vi "IMAQ subtract background.vi"(7 "FakeCamera in":refnum<class "Point Grey Camera.lvclass">, 8 "error in (no error)":errorcluster, 11 "Image in":T1) -> (0 "error out":errorcluster, 1 "Intensity Graph":u16[][](graph), 2 "Line Graph 2":cluster{"x0":sgl, "dx":sgl, "Pixels Line":sgl[]} {"dx" format="%.2f"; "x0" format="%.2f"}, 3 "Refnum out":T1, 4 "Line Graph":cluster{"x0":sgl, "dx":sgl, "Pixels Line":sgl[]} {"dx" format="%.2f"; "x0" format="%.2f"}, 5 "FakeCamera out":refnum<class "Point Grey Camera.lvclass">)   [LabVIEW 2020, in "Point Grey Camera.lvclass"]
uses:
  Point Grey Camera.lvclass
  IMAQ Image.ctl
  Point Grey Camera.lvclass/Point Grey Camera.ctl
  NI_Vision_Development_Module.lvlib
  NI_AALBase.lvlib
panel:
  out "create BG":u32
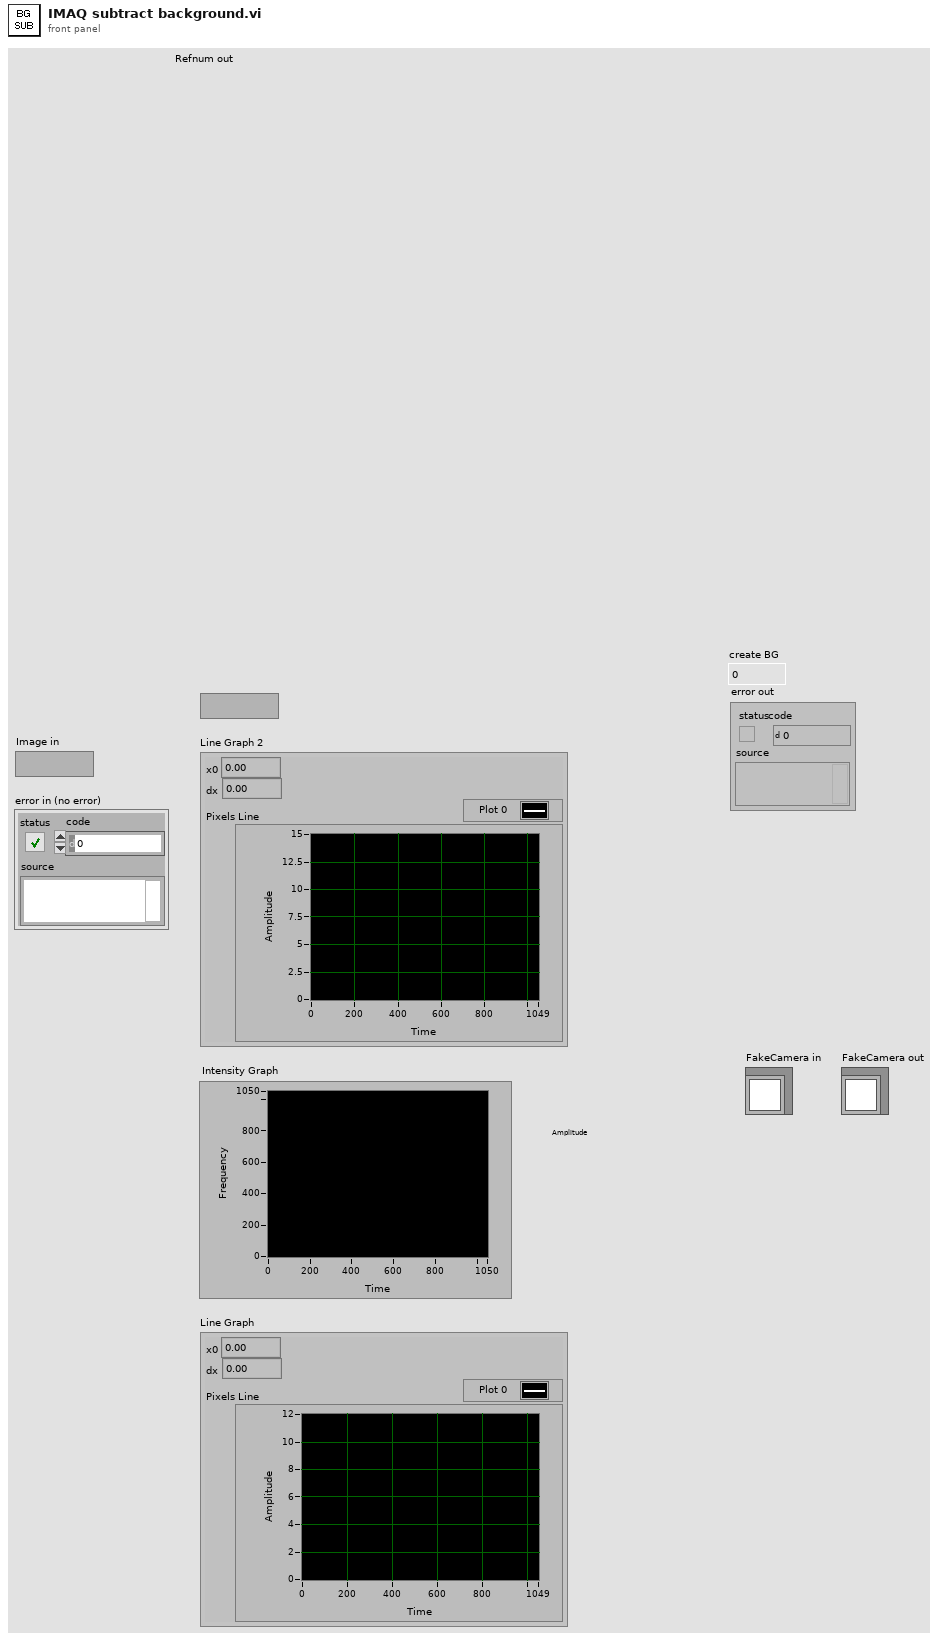
[diagram p1: front panel]
types:
  T1 = typedef "IMAQ Image.ctl" = refnum<image>
  T2 = cluster{"X Size":i32, "Y Size":i32, "% Tolerance":i32}
  T3 = typedef "ROI Descriptor" = cluster{"Global Rectangle":i32[], "Contours":cluster{"ID":enum32{"External", "Internal"}, "Type":u32, "Coordinates":i32[]}[]}
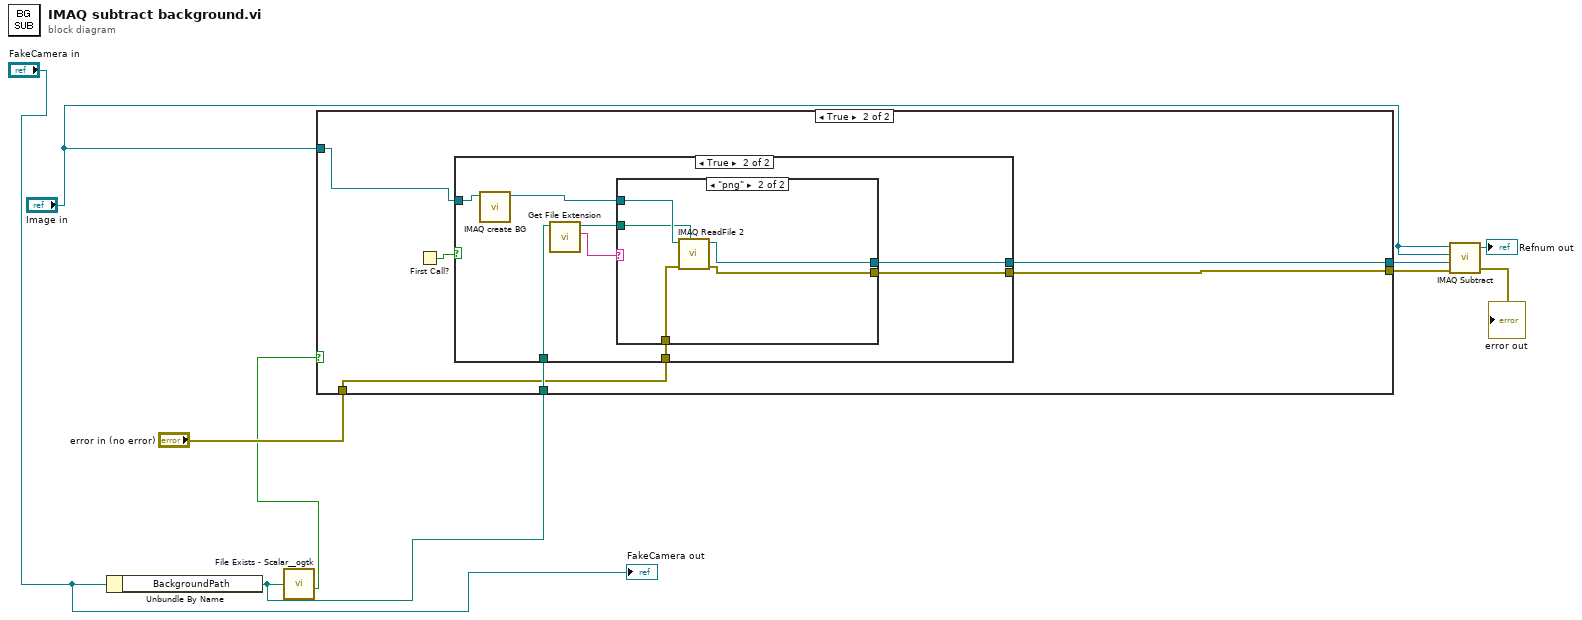
[diagram p0: block diagram]
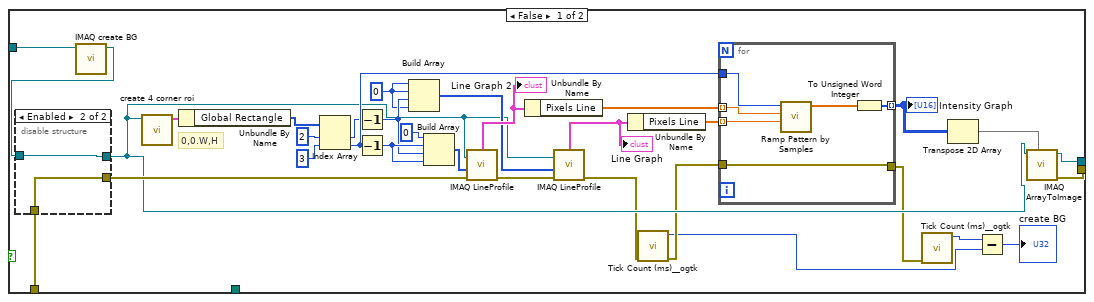
[diagram p2: hidden frame]
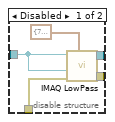
[diagram p3: hidden frame]
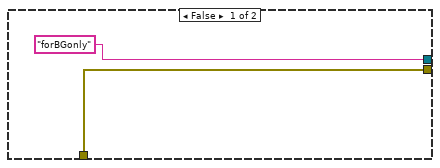
[diagram p4: hidden frame]
diagram:
  n1 = Unbundle By Name("FakeCamera in") -> ("BackgroundPath"=w3:path)
  n2 = call "File Exists - Scalar__ogtk.vi"("file path"=w3) -> ("exists"=w5:bool)  [unwired: 6 in, 1 out]
  n3 = case shown="True" w5 {
    tunnel: "error in (no error)" -> [w40 w56]
    tunnel: [w39 w55] -> w7
    tunnel: [w36 w57] -> w6
    tunnel: "Image in" -> [w11 w59]
    tunnel: w3 -> [_ w58]
    frame False {
      w28 = 0 ("element")
      # "0,0.W,H"
      n4 = call "IMAQ create BG.vi"("Refnum in"=w11) -> ("Refnum out"=w10:T1)  [unwired: 10 in]
      n5 = disable-structure shown="Enabled" {
        disable-tunnel: w10 -> [w46 w48]
        disable-tunnel: w40 -> [w45 w47]
        disable-tunnel: [w44 w47] -> w37
        disable-tunnel: [w42 w48] -> w18
        frame Disabled {
          n6 = call "IMAQ LowPass"("Image Src"=w46, "Size & Tolerance"=T2 {"X Size"=7, "Y Size"=7, "% Tolerance"=10}, "Image Dst"=w46, "error in (no error)"=w45) -> ("Image Dst Out"=w42:T1, "error out"=w44:errorcluster)  [unwired: 3 in]
        }
        frame Enabled {
        }
      }
      n7 = call "create 4 corner roi.vi"("Refnum in"=w18) -> ("ROI Descriptor"=w41:T3)  [unwired: 9 in, 1 out]
      n8 = Unbundle By Name(w41) -> ("Global Rectangle"=w19:i32[])
      n9 = Index Array(array=w19, index #1=2 ("index"), index #2=3 ("index")) -> (element #1=w31:i32, element #2=w33:i32)
      n10 = Decrement(x=w31) -> (x-1=w30:i32)
      n11 = Decrement(x=w33) -> (x-1=w32:i32)
      n12 = Build Array(w28, w28, w30, w28) -> (w22:i32[])
      n13 = Build Array(0 ("element"), w32, w30, w32) -> (w23:i32[])
      n14 = call "IMAQ LineProfile"("error in (no error)"=w37, "Line Coordinates"=w23, "Image"=w18) -> ("error out"=w38:errorcluster, "Line Graph"=w25:cluster{"x0":sgl, "dx":sgl, "Pixels Line":sgl[]})  [unwired: 2 in, 2 out]
      "Line Graph 2" <- w25
      n15 = Unbundle By Name(w25) -> ("Pixels Line"=w27:sgl[])
      n16 = call "IMAQ LineProfile"("error in (no error)"=w38, "Line Coordinates"=w22, "Image"=w18) -> ("error out"=w17:errorcluster, "Line Graph"=w24:cluster{"x0":sgl, "dx":sgl, "Pixels Line":sgl[]})  [unwired: 2 in, 2 out]
      "Line Graph" <- w24
      n17 = Unbundle By Name(w24) -> ("Pixels Line"=w26:sgl[])
      n18 = call "Tick Count (ms)__ogtk.vi"("error in (no error)"=w17) -> ("error out"=w16:errorcluster, "millisecond timer value"=w13:u32)  [unwired: 9 in]
      n19 = for {
        tunnel: w26 -> [w52] mode=indexing
        tunnel: w27 -> [w53] mode=indexing
        tunnel: w33 -> [w54]
        tunnel: [w50] -> w34 mode=indexing
        tunnel: w16 -> [w49]
        tunnel: [w49] -> w15
        n20 = call "Ramp Pattern by Samples.vi"("start"=w52, "end"=w53, "samples"=w54) -> ("Ramp Pattern"=w51:dbl[])  [unwired: 7 in, 1 out]
        n21 = To Unsigned Word Integer(number=w51) -> (unsigned 16bit integer=w50:u16[])
      }
      "Intensity Graph" <- w34
      n22 = call "Tick Count (ms)__ogtk.vi"("error in (no error)"=w15) -> ("millisecond timer value"=w14:u32)  [unwired: 9 in, 1 out]
      n23 = Transpose 2D Array(2D array=w34) -> (transposed array=w35:u16[][])
      n24 = Subtract(x=w14, y=w13) -> (x-y=→"create BG":u32)
      n25 = call "IMAQ ArrayToImage"("Image Pixels (U16)"=w35, "Image"=w18) -> ("error out"=w39:errorcluster, "Image Out"=w36:T1)  [unwired: 8 in]
    }
    frame True {
      n26 = First Call?() -> (First Call?: T/F=w60:bool)
      n27 = case shown="True" w60 {
        tunnel: w59 -> [_ w70]
        tunnel: w58 -> [_ w69]
        tunnel: ["forBGonly" ("Image Name") w66] -> w57
        tunnel: w56 -> [w62 w65]
        tunnel: [w62 w64] -> w55
        frame False {
        }
        frame True {
          n28 = call "IMAQ create BG.vi"("Refnum in"=w70) -> ("Refnum out"=w67:T1)  [unwired: 10 in]
          n29 = call "Get File Extension.vi"("file"=w69) -> ("lowercase file extension"=w68:string, "dup file"=w63:path)  [unwired: 6 in, 3 out]
          n30 = case shown="\"png\"" w68 {
            tunnel: w67 -> [w72 w77]
            tunnel: [w72 w76] -> w66
            tunnel: w65 -> [w71 w75]
            tunnel: [w71 w74] -> w64
            tunnel: w63 -> [_ w73]
            frame "False", Default {
            }
            frame "png" {
              n31 = call "IMAQ ReadFile 2"("File Path"=w73, "error in (no error)"=w75, "Image"=w77) -> ("error out"=w74:errorcluster, "Image Out"=w76:T1)  [unwired: 4 in, 3 out]
            }
          }
        }
      }
    }
  }
  n32 = call "IMAQ Subtract"("Image Src A"="Image in", "Image Dst"="Image in", "Image Src B"=w6, "error in (no error)"=w7) -> ("Image Dst Out"=→"Refnum out":T1, "error out"=→"error out":errorcluster)  [unwired: 3 in]
  "FakeCamera out" <- "FakeCamera in"
